vi "MeasureAtFreq.vi"(8 "error in (no error)":errorcluster, 10 "Frequency (Hz)":dbl, 11 "NetA_RSZVL in":refnum<class "NetA_RSZVL.lvclass">) -> (0 "error out":errorcluster, 2 "Power (dBm)":dbl, 3 "NetA_RSZVL out":refnum<class "NetA_RSZVL.lvclass">)   [LabVIEW 2014, in "NetA_RSZVL.lvclass"]
uses:
  NetA_RSZVL.lvclass
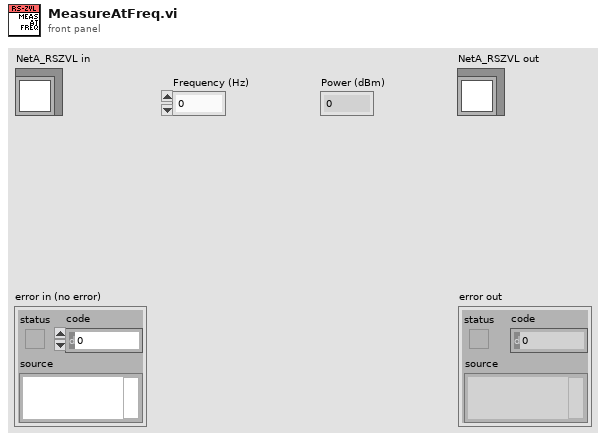
[diagram p1: front panel]
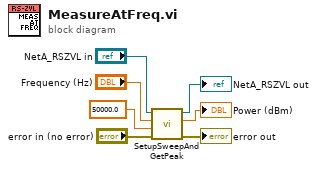
[diagram p0: block diagram]
diagram:
  n1 = call-dynamic "SetupSweepAndGetPeak.vi"("error in (no error)"="error in (no error)", "Span(Hz)"=50000.0, "Center Frequency(Hz)"="Frequency (Hz)", "NetA_RSZVL in"="NetA_RSZVL in") -> ("error out"=→"error out":errorcluster, "Calibrated Amplitude (dBm)"=→"Power (dBm)":dbl, "NetA_RSZVL out"=→"NetA_RSZVL out":refnum<class "NetA_RSZVL.lvclass">)  [unwired: 4 in, 1 out]
